vi "AIT 664 - Read Tx Ports XML.vi"(0 "Refnum in":refnum<k20>, 11 "error in (no error)":errorcluster) -> (4 "Tx Message Port":T1, 15 "error out":errorcluster)   [LabVIEW 2013, in "AIT 664 Custom Device.lvlib"]
doc: "Read TxMessagePort xml"
uses:
  AIT 664 Custom Device.lvlib
  Controls/664 - XML Tx Message Port.ctl
  Controls/664 - Sampling Type.ctl
  Controls/664 -Param.ctl
  <vilib>/xml/Close Reference(NNMap).vi
  <vilib>/xml/Close Reference(Node).vi
  <resource>/objmgr/DOMUserDefRef.rc
  <vilib>/xml/NI_XML.lvlib
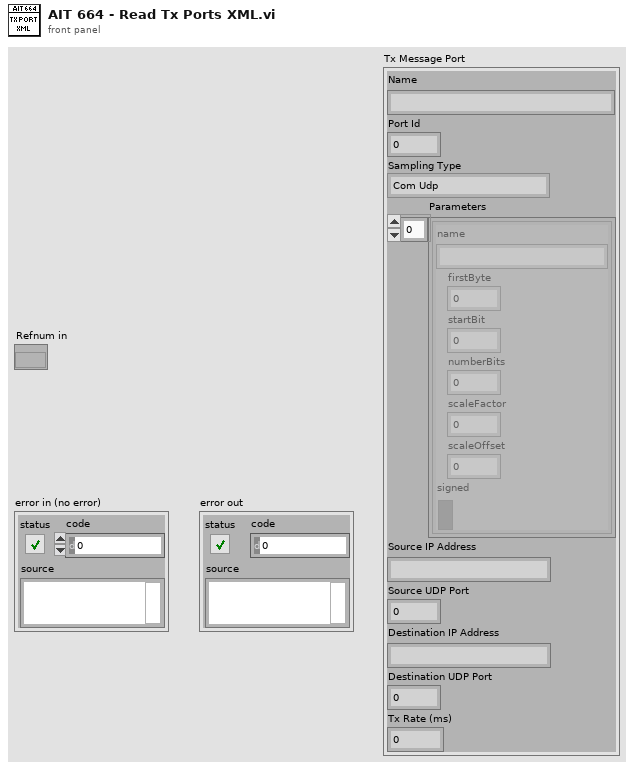
[diagram p1: front panel]
types:
  T1 = typedef "AIT 664 Custom Device.lvlib/664 - XML Tx Message Port.ctl" = cluster{"Name":string, "Port Id":u32, "Sampling Type":T2, "Parameters":T3[], "Source IP Address":string, "Source UDP Port":u32, "Destination IP Address":string, "Destination UDP Port":u32, "Tx Rate (ms)":u32}
  T2 = typedef "AIT 664 Custom Device.lvlib/664 - Sampling Type.ctl" = enum16{"Com Udp", "Com Udp Queuing", "Sap Udp", "Sap Ip", "Sap Mac", "Unknown"}
  T3 = typedef "AIT 664 Custom Device.lvlib/664 -Param.ctl" = cluster{"name":string, "firstByte":i32, "startBit":i32, "numberBits":i32, "scaleFactor":dbl, "scaleOffset":dbl, "signed":bool}
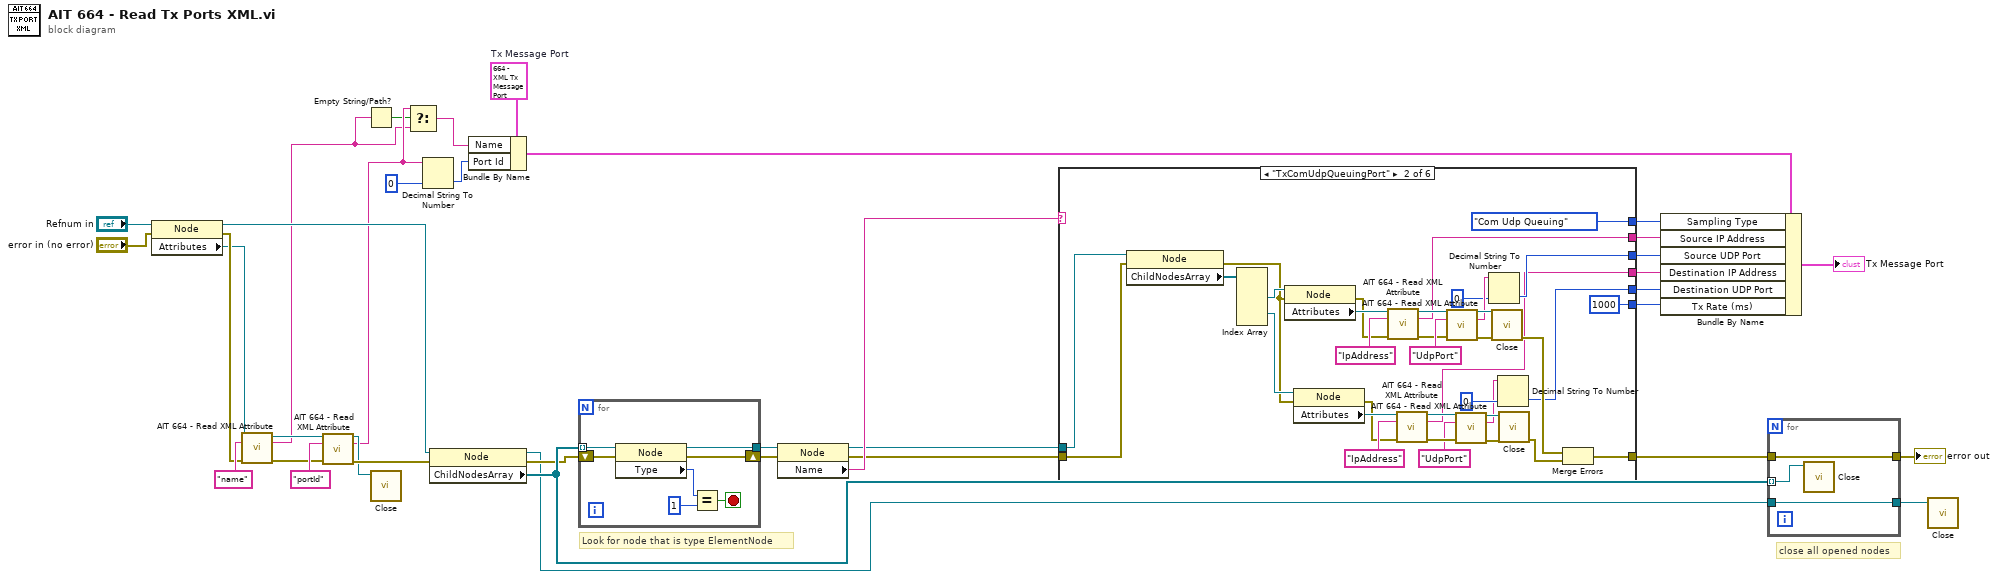
[diagram p0: block diagram]
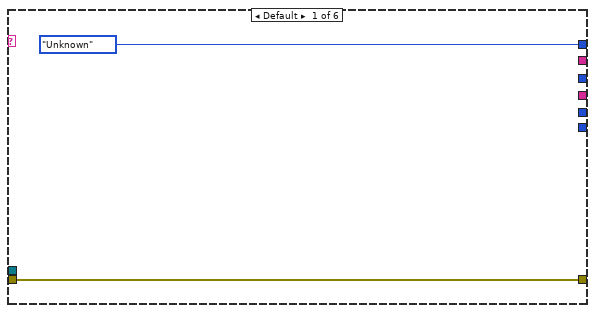
[diagram p2: hidden frame]
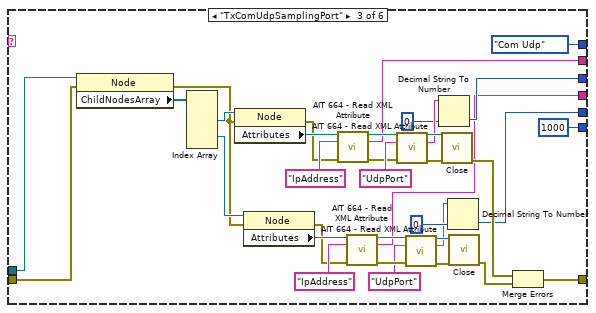
[diagram p3: hidden frame]
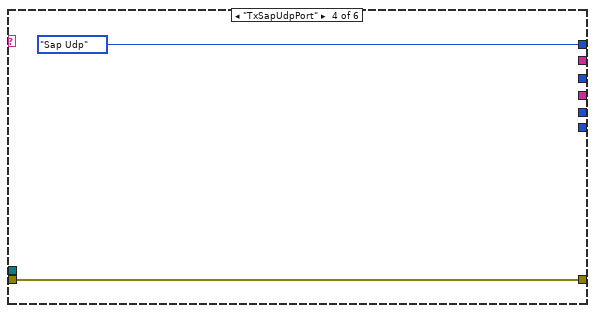
[diagram p4: hidden frame]
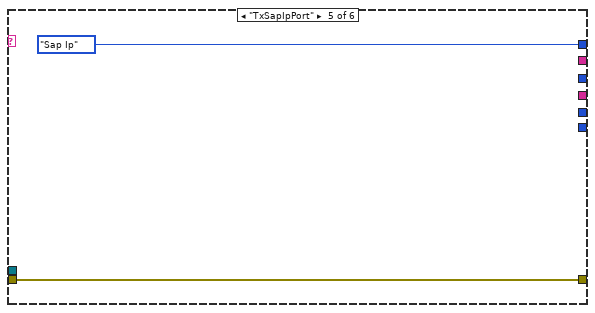
[diagram p5: hidden frame]
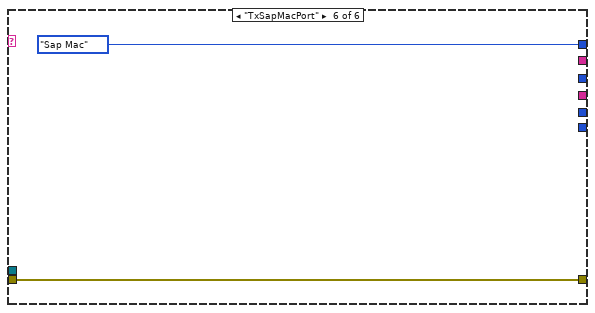
[diagram p6: hidden frame]
diagram:
  w27 = T1 {"Name"="", "Port Id"=0, "Sampling Type"=enum."Com Udp", "Parameters"=[], "Source IP Address"="", "Source UDP Port"=0, "Destination IP Address"="", "Destination UDP Port"=0, "Tx Rate (ms)"=0}  # Tx Message Port
  # "close all opened nodes"
  # "Look for node that is type ElementNode"
  n1 = property class="Node"(reference="Refnum in", error in="error in (no error)") -> (reference out=w28:refnum<k20>, error out=w19:errorcluster, "Attributes"=w18:refnum<k20>)
  n2 = call "AIT 664 - Read XML Attribute.vi"("Attributes In"=w18, "Attribute Name"="name", "error in (no error)"=w19) -> ("Attributes Out"=w22:refnum<k20>, "Attribute Text"=w2:string, "error out"=w21:errorcluster)  [unwired: 10 in]
  n3 = call "AIT 664 - Read XML Attribute.vi"("Attributes In"=w22, "Attribute Name"="portId", "error in (no error)"=w21) -> ("Attributes Out"=w24:refnum<k20>, "Attribute Text"=w5:string, "error out"=w29:errorcluster)  [unwired: 10 in]
  n4 = Empty String/Path?(string/path=w2) -> (empty?=w3:bool)
  n5 = call-poly <vilib>:"Close.vi"("named node map"=w24) -> ()  [unwired: 8 in, 1 out]
  n6 = Select(t=w5, s=w3, f=w2) -> (s? t:f=w4:string)
  n7 = Decimal String To Number(string=w5, default (0L)=u32 0 ("default (0 I32)")) -> (number=w26:u32)  [unwired: 1 in, 1 out]
  n8 = property class="Node"(reference=w28, error in=w29) -> (reference out=w15:refnum<k20>, error out=w34:errorcluster, "ChildNodesArray"=w37:refnum<k20>[])
  n9 = Bundle By Name(cluster=w27, "Name"=w4, "Port Id"=w26) -> (w30:T1)
  n10 = for {
    tunnel: w37 -> [w44] mode=indexing
    tunnel: [w40] -> w33
    shift-right: [w38] -> w35
    shift-left: w34 -> [w39]
    stop <- w43 stop-if-true
    n11 = property class="Node"(reference=w44, error in=w39) -> (reference out=w40:refnum<k20>, error out=w38:errorcluster, "Type"=w41:i32)
    n12 = Equal?(x=w41, y=1) -> (x = y?=w43:bool)
  }
  n13 = property class="Node"(reference=w33, error in=w35) -> (reference out=w10:refnum<k20>, error out=w11:errorcluster, "Name"=w36:string)
  n14 = case shown="\"TxComUdpQueuingPort\"" w36 {
    tunnel: [664_-_Sampling_Type."Unknown" ("Sampling Type") 664_-_Sampling_Type."Com Udp Queuing" ("Sampling Type") 664_-_Sampling_Type."Com Udp" ("Sampling Type") 664_-_Sampling_Type."Sap Udp" ("Sampling Type") 664_-_Sampling_Type."Sap Ip" ("Sampling Type") 664_-_Sampling_Type."Sap Mac" ("Sampling Type")] -> w31
    tunnel: w11 -> [w45 w53 w89 w117 w119 w121]
    tunnel: [w45 w52 w88 w117 w119 w121] -> w12
    tunnel: w10 -> [_ w59 w95 _ _ _]
    tunnel: [_ w51 w87 _ _ _] -> w9
    tunnel: [_ w50 w86 _ _ _] -> w8
    tunnel: [_ w49 w85 _ _ _] -> w7
    tunnel: [_ w48 w84 _ _ _] -> w6
    tunnel: [_ u32 1000 ("Tx Rate (ms)") u32 1000 ("Tx Rate (ms)") _ _ _] -> w1
    frame Default {
    }
    frame "TxComUdpQueuingPort" {
      n15 = property class="Node"(reference=w59, error in=w53) -> (error out=w57:errorcluster, "ChildNodesArray"=w67:refnum<k20>[])  [unwired: 1 out]
      n16 = Index Array(array=w67) -> (element #2=w79:refnum<k20>, element #4=w80:refnum<k20>)  [unwired: 5 in, 3 out]
      n17 = property class="Node"(reference=w79, error in=w57) -> (error out=w58:errorcluster, "Attributes"=w60:refnum<k20>)  [unwired: 1 out]
      n18 = property class="Node"(reference=w80, error in=w57) -> (error out=w56:errorcluster, "Attributes"=w74:refnum<k20>)  [unwired: 1 out]
      n19 = call "AIT 664 - Read XML Attribute.vi"("Attributes In"=w60, "Attribute Name"="IpAddress", "error in (no error)"=w58) -> ("Attributes Out"=w62:refnum<k20>, "Attribute Text"=w51:string, "error out"=w63:errorcluster)  [unwired: 10 in]
      n20 = call "AIT 664 - Read XML Attribute.vi"("Attributes In"=w74, "Attribute Name"="IpAddress", "error in (no error)"=w56) -> ("Attributes Out"=w72:refnum<k20>, "Attribute Text"=w49:string, "error out"=w71:errorcluster)  [unwired: 10 in]
      n21 = call "AIT 664 - Read XML Attribute.vi"("Attributes In"=w62, "Attribute Name"="UdpPort", "error in (no error)"=w63) -> ("Attributes Out"=w76:refnum<k20>, "Attribute Text"=w66:string, "error out"=w75:errorcluster)  [unwired: 10 in]
      n22 = call "AIT 664 - Read XML Attribute.vi"("Attributes In"=w72, "Attribute Name"="UdpPort", "error in (no error)"=w71) -> ("Attributes Out"=w78:refnum<k20>, "Attribute Text"=w68:string, "error out"=w77:errorcluster)  [unwired: 10 in]
      n23 = Decimal String To Number(string=w66, default (0L)=u32 0 ("default (0 I32)")) -> (number=w50:u32)  [unwired: 1 in, 1 out]
      n24 = call-poly <vilib>:"Close.vi"("error in (no error)"=w75, "named node map"=w76) -> ("error out"=w55:errorcluster)  [unwired: 7 in]
      n25 = Decimal String To Number(string=w68, default (0L)=u32 0 ("default (0 I32)")) -> (number=w48:u32)  [unwired: 1 in, 1 out]
      n26 = call-poly <vilib>:"Close.vi"("error in (no error)"=w77, "named node map"=w78) -> ("error out"=w54:errorcluster)  [unwired: 7 in]
      n27 = Merge Errors(w55, w54) -> (w52:errorcluster)
    }
    frame "TxComUdpSamplingPort" {
      n28 = property class="Node"(reference=w95, error in=w89) -> (error out=w93:errorcluster, "ChildNodesArray"=w103:refnum<k20>[])  [unwired: 1 out]
      n29 = Index Array(array=w103) -> (element #2=w115:refnum<k20>, element #4=w116:refnum<k20>)  [unwired: 5 in, 3 out]
      n30 = property class="Node"(reference=w115, error in=w93) -> (error out=w94:errorcluster, "Attributes"=w96:refnum<k20>)  [unwired: 1 out]
      n31 = property class="Node"(reference=w116, error in=w93) -> (error out=w92:errorcluster, "Attributes"=w110:refnum<k20>)  [unwired: 1 out]
      n32 = call "AIT 664 - Read XML Attribute.vi"("Attributes In"=w96, "Attribute Name"="IpAddress", "error in (no error)"=w94) -> ("Attributes Out"=w98:refnum<k20>, "Attribute Text"=w87:string, "error out"=w99:errorcluster)  [unwired: 10 in]
      n33 = call "AIT 664 - Read XML Attribute.vi"("Attributes In"=w110, "Attribute Name"="IpAddress", "error in (no error)"=w92) -> ("Attributes Out"=w108:refnum<k20>, "Attribute Text"=w85:string, "error out"=w107:errorcluster)  [unwired: 10 in]
      n34 = call "AIT 664 - Read XML Attribute.vi"("Attributes In"=w98, "Attribute Name"="UdpPort", "error in (no error)"=w99) -> ("Attributes Out"=w112:refnum<k20>, "Attribute Text"=w102:string, "error out"=w111:errorcluster)  [unwired: 10 in]
      n35 = call "AIT 664 - Read XML Attribute.vi"("Attributes In"=w108, "Attribute Name"="UdpPort", "error in (no error)"=w107) -> ("Attributes Out"=w114:refnum<k20>, "Attribute Text"=w104:string, "error out"=w113:errorcluster)  [unwired: 10 in]
      n36 = Decimal String To Number(string=w102, default (0L)=u32 0 ("default (0 I32)")) -> (number=w86:u32)  [unwired: 1 in, 1 out]
      n37 = call-poly <vilib>:"Close.vi"("error in (no error)"=w111, "named node map"=w112) -> ("error out"=w91:errorcluster)  [unwired: 7 in]
      n38 = Decimal String To Number(string=w104, default (0L)=u32 0 ("default (0 I32)")) -> (number=w84:u32)  [unwired: 1 in, 1 out]
      n39 = call-poly <vilib>:"Close.vi"("error in (no error)"=w113, "named node map"=w114) -> ("error out"=w90:errorcluster)  [unwired: 7 in]
      n40 = Merge Errors(w91, w90) -> (w88:errorcluster)
    }
    frame "TxSapUdpPort" {
    }
    frame "TxSapIpPort" {
    }
    frame "TxSapMacPort" {
    }
  }
  n41 = Bundle By Name(cluster=w30, "Sampling Type"=w31, "Source IP Address"=w9, "Source UDP Port"=w8, "Destination IP Address"=w7, "Destination UDP Port"=w6, "Tx Rate (ms)"=w1) -> (→"Tx Message Port":T1)
  n42 = for {
    tunnel: w12 -> [w124]
    tunnel: w37 -> [w125] mode=indexing
    tunnel: [w124] -> w13
    tunnel: w15 -> [w123]
    tunnel: [w123] -> w14
    n43 = call-poly <vilib>:"Close.vi"("node"=w125) -> ()  [unwired: 8 in, 1 out]
  }
  "error out" <- w13
  n44 = call-poly <vilib>:"Close.vi"("node"=w14) -> ()  [unwired: 8 in, 1 out]
